vi "Init Actor Queues FOR TESTING ONLY.vi"(8 "error in (no error)":errorcluster, 10 "Actor-To-Caller Enqueuer":refnum<class "Message Enqueuer.lvclass">, 11 "Actor in":refnum<class "Actor.lvclass">) -> (0 "error out":errorcluster, 1 "Actor-To-Self Dequeuer":refnum<class "Message Dequeuer.lvclass">, 2 "Actor-To-Self Enqueuer":refnum<class "Message Enqueuer.lvclass">, 3 "Actor out":refnum<class "Actor.lvclass">)   [LabVIEW 2020, in "Actor Framework.lvlib"]
doc: "<p>Provides access the To-Self and To-Caller message queues for an actor without launching the actor.</p>\n\n<p>Use this VI to test how an actor handles messages. Do not use this VI in code that you deploy.</p>"
uses:
  Actor Framework.lvlib
  Message Priority Queue/Message Priority Queue.lvclass
  Actor.lvclass
  Message Dequeuer/Message Dequeuer.lvclass
  Message Enqueuer/Message Enqueuer.lvclass
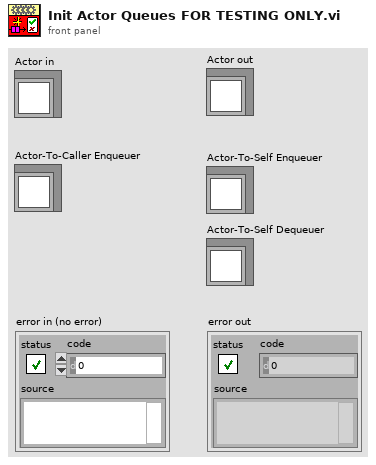
[diagram p1: front panel]
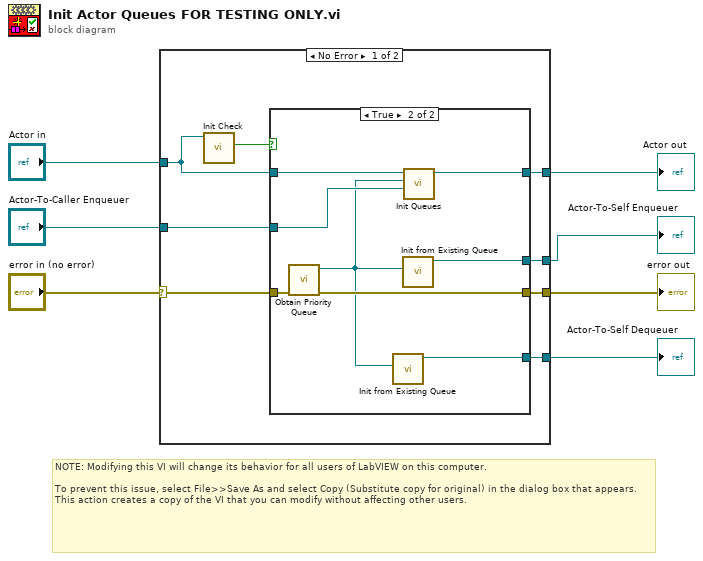
[diagram p0: block diagram]
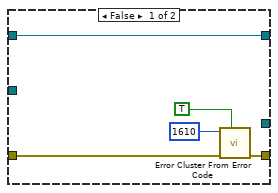
[diagram p2: hidden frame]
diagram:
  # "NOTE: Modifying this VI will change its behavior for all users of LabVIEW on this computer.\n\nTo prevent this issue, select File>>Save As and select Copy (Substitute copy for original) in the dialog box that appears. This action creates a copy of the VI that you can modify without affecting other users."
  n1 = case shown="No Error" "error in (no error)" {
    selector: "error in (no error)" -> [w13 w30]
    tunnel: "Actor in" -> [w11 w29]
    tunnel: [w15 w29] -> w5
    tunnel: "Actor-To-Caller Enqueuer" -> [w14 _]
    tunnel: [w12 w30] -> w3
    tunnel: [w10 _] -> w2
    tunnel: [w9 _] -> w1
    frame No Error {
      n2 = call "Init Check.vi"("Actor in"=w11) -> ("Not initialized?"=w8:bool)  [unwired: 10 in]
      n3 = case shown="True" w8 {
        tunnel: [w20 w24] -> w15
        tunnel: w14 -> [_ w23]
        tunnel: w13 -> [w19 w28]
        tunnel: w11 -> [w20 w25]
        tunnel: [w18 w27] -> w12
        tunnel: [_ w26] -> w10
        tunnel: [_ w21] -> w9
        frame False {
          n4 = call <vilib>:"Error Cluster From Error Code.vi"("show call chain? (False)"=TRUE, "error in (no error)"=w19, "error code (0)"=1610) -> ("error out"=w18:errorcluster)  [unwired: 6 in]
        }
        frame True {
          n5 = call "Obtain Priority Queue.vi"("error in (no error)"=w28) -> ("error out"=w27:errorcluster, "Priority Queue"=w22:refnum<class "Message Priority Queue.lvclass">)  [unwired: 9 in]
          n6 = call "Init from Existing Queue.vi"("Priority Queue"=w22) -> ("Message Dequeuer"=w26:refnum<class "Message Dequeuer.lvclass">)  [unwired: 10 in]
          n7 = call "Init from Existing Queue.vi"("Priority Queue"=w22) -> ("Message Enqueuer"=w21:refnum<class "Message Enqueuer.lvclass">)  [unwired: 10 in]
          n8 = call "Init Queues.vi"("Self-To-Caller"=w23, "Self-ToSelf"=w22, "Actor in"=w25) -> ("Actor out"=w24:refnum<class "Actor.lvclass">)  [unwired: 8 in]
        }
      }
    }
    frame Error {
    }
  }
  "Actor out" <- w5
  "error out" <- w3
  "Actor-To-Self Enqueuer" <- w1
  "Actor-To-Self Dequeuer" <- w2
